vi "DAQ_TTC Meas Configure and Measure.vi"(0 "DAQmx Task In":refnum<k21>, 2 "Execution Option":T7, 5 "Range and Terminal Settings":T1={"Global Settings"={"Min Temp (deg C)"=0.0, "Max Temp (deg C)"=100.0, "Thermocouple Type"=10072, "CJC Temp (deg C)"=25.0, "Enable Autozero"=FALSE, "Auto Zero Mode"=10230}, "Specific Channel Settings"=[]} {"Specific Channel Settings"."Thermocouple Type" items=["J"=10072, "K"=10073, "N"=10077, "R"=10082, "S"=10085, "T"=10086, "B"=10047, "E"=10055]; "Global Settings"."Auto Zero Mode" items=["None"=10230, "Once"=10244, "Every Sample"=10164]; "Global Settings"."Thermocouple Type" items=["J"=10072, "K"=10073, "N"=10077, "R"=10082, "S"=10085, "T"=10086, "B"=10047, "E"=10055]; "Global Settings"."CJC Temp (deg C)" format="%.2f"; "Global Settings"."Min Temp (deg C)" format="%.2f"; "Global Settings"."Max Temp (deg C)" format="%.2f"}, 7 "Timing and Trigger Settings":T3={"Timing Settings"={"Sample Clock Source"="OnboardClock", "Sample Rate(Hz)"=100.0, "Number of Samples"=10, "Sample Timing Engine"=enum."Auto"}, "Trigger Settings"={"Trigger Type"=enum."No Trigger", "Digital Start Trigger Source"="", "Digital Start Trigger Edge"=10280}} {"Trigger Settings"."Digital Start Trigger Edge" items=["Rising"=10280, "Falling"=10171]; "Timing Settings"."Sample Rate(Hz)" format="%.2p"}, 11 "error in":errorcluster) -> (4 "DAQmx Task Out":refnum<k21>, 6 "Temperature Waveforms":waveform(dbl)[](graph), 8 "Temperature Measurements":T6 {"Average Temperature(K)" format="%.2p"; "Average Temperature(deg C)" format="%.2p"}, 10 "Acquisition Time (s)":dbl=0.1 format="%.2p", 15 "error out":errorcluster)   [LabVIEW 2021, in "DAQ_Temperature Thermocouple Measurement.lvlib"]
doc: "Configure, initiate and fetch temperature thermocouple measurements from the channels configured."
uses:
  DAQ_Temperature Thermocouple Measurement.lvlib
  Common/Typedefs/Execution Options - Measure.ctl
  Typedefs/Temperature Thermocouple Measurements.ctl
  Typedefs/Timing & Trigger Settings.ctl
  Typedefs/Timing Settings.ctl
  Typedefs/Trigger Settings.ctl
  Typedefs/Range and Terminal Settings.ctl
  Typedefs/Specific Channel Settings.ctl
  <vilib>/DAQmx/read.llb/DAQmx Read (Analog 1D Wfm NChan NSamp).vi
  <vilib>/DAQmx/configure/timing.llb/DAQmx Timing (Sample Clock).vi
  <vilib>/DAQmx/configure/trigger.llb/DAQmx Start Trigger (Digital Edge).vi
  <vilib>/DAQmx/miscellaneous.llb/DAQmx Fill In Error Info.vi
  <resource>/objmgr/daqmx.rc
panel:
  # "Outputs"
  # "Inputs"
  # "Physical Channel Name"
  # "Thermocouple Type"
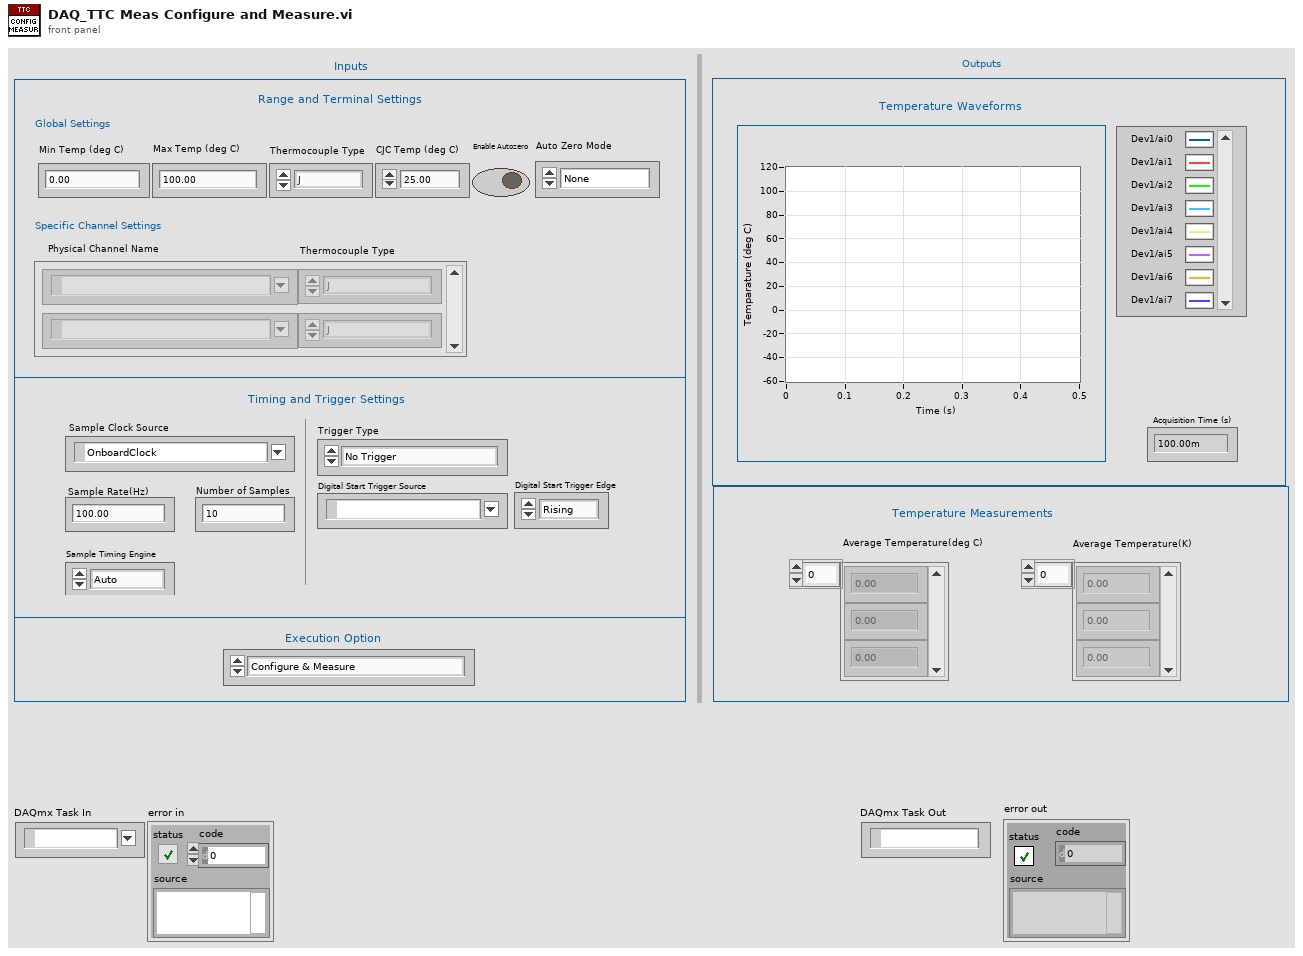
[diagram p1: front panel]
types:
  T1 = typedef "DAQ_Temperature Thermocouple Measurement.lvlib/Range and Terminal Settings.ctl" = cluster{"Global Settings":cluster{"Min Temp (deg C)":dbl, "Max Temp (deg C)":dbl, "Thermocouple Type":i32, "CJC Temp (deg C)":dbl, "Enable Autozero":bool, "Auto Zero Mode":i32}, "Specific Channel Settings":T2[]}
  T2 = typedef "DAQ_Temperature Thermocouple Measurement.lvlib/Specific Channel Settings.ctl" = cluster{"Physical Channel Name":tag, "Thermocouple Type":i32}
  T3 = typedef "DAQ_Temperature Thermocouple Measurement.lvlib/Timing & Trigger Settings.ctl" = cluster{"Timing Settings":T4, "Trigger Settings":T5}
  T4 = typedef "DAQ_Temperature Thermocouple Measurement.lvlib/Timing Settings.ctl" = cluster{"Sample Clock Source":tag, "Sample Rate(Hz)":dbl, "Number of Samples":i32, "Sample Timing Engine":enum16{"te0", "te1", "ai", "Auto"}}
  T5 = typedef "DAQ_Temperature Thermocouple Measurement.lvlib/Trigger Settings.ctl" = cluster{"Trigger Type":enum16{"No Trigger", "Digital Start"}, "Digital Start Trigger Source":tag, "Digital Start Trigger Edge":i32}
  T6 = typedef "DAQ_Temperature Thermocouple Measurement.lvlib/Temperature Thermocouple Measurements.ctl" = cluster{"Average Temperature(deg C)":dbl[], "Average Temperature(K)":dbl[]}
  T7 = typedef "Execution Options - Measure.ctl" = enum16{"Configure & Measure", "Configure only", "Measure only"}
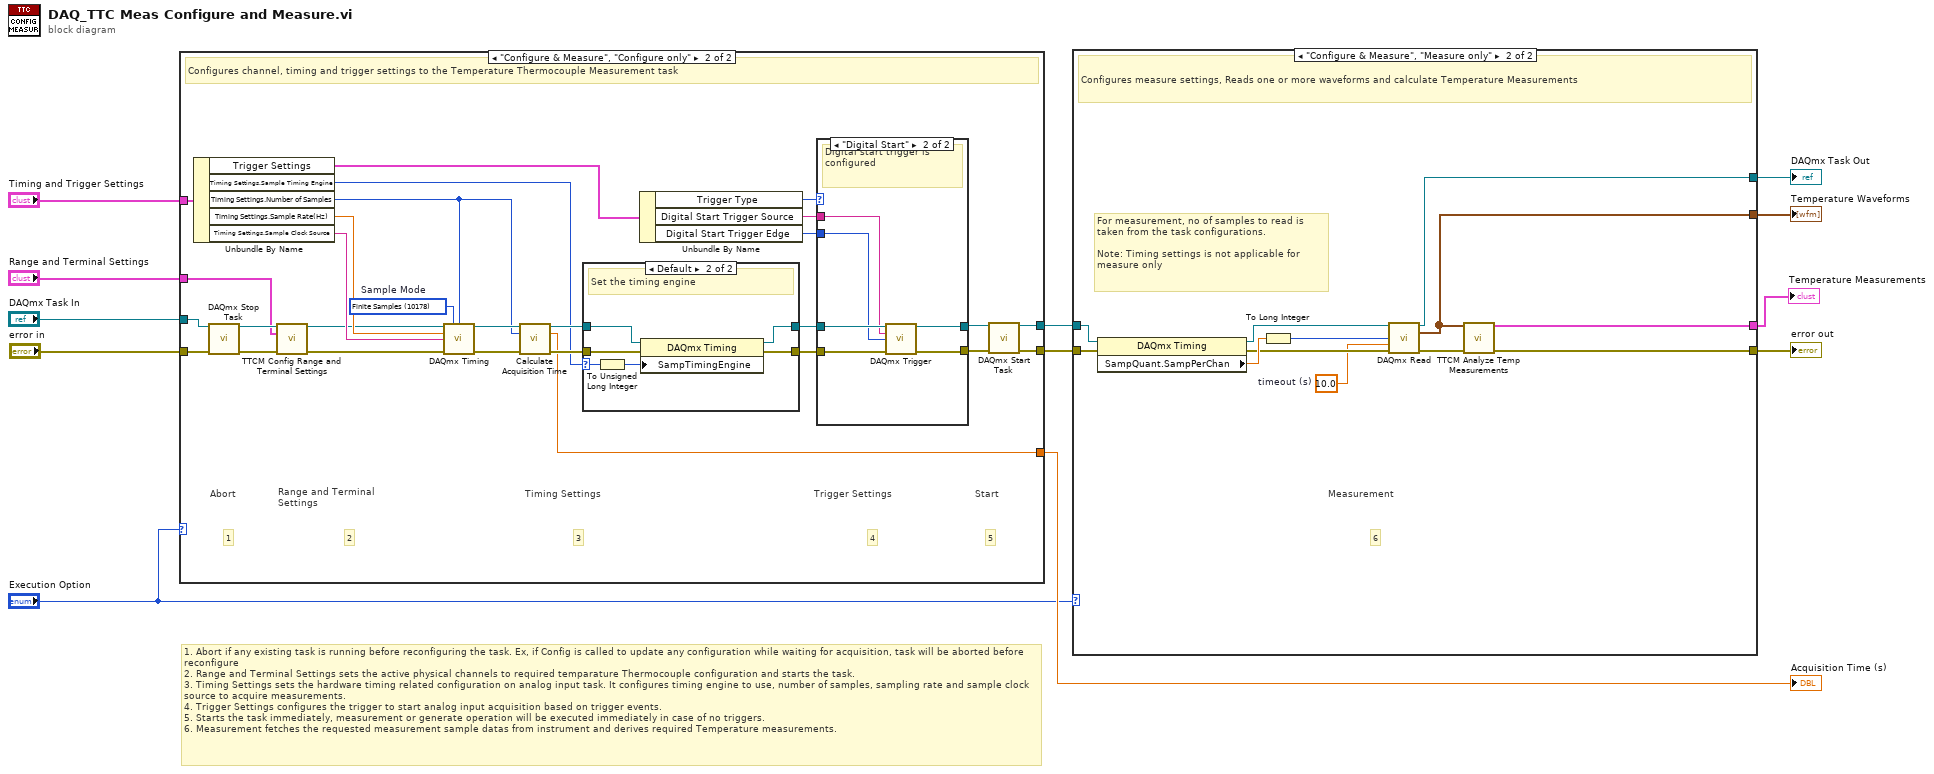
[diagram p0: block diagram]
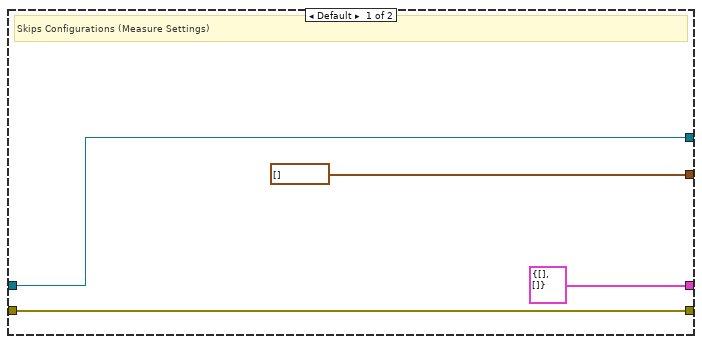
[diagram p5: hidden frame]
diagram:
  # "1. Abort if any existing task is running before reconfiguring the task. Ex, if Config is called to update any configuration while waiting for acquisition, task will be aborted before reconfigure\n2. Range and Terminal Settings sets the active physical channels to required temparature Thermocouple configuration and starts the task.\n3. Timing Settings sets the hardware timing related configuration on analog input task. It configures timing engine to use, number of samples, sampling rate and sample clock source to acquire measurements.\n4. Trigger Settings configures the trigger to start analog input acquisition based on trigger events.\n5. Starts the task immediately, measurement or generate operation will be executed immediately in case of no triggers.\n6. Measurement fetches the requested measurement sample datas from instrument and derives required Temperature measurements."
  n1 = case shown="\"Configure & Measure\", \"Configure only\"" "Execution Option" {
    tunnel: "error in" -> [w14 w19]
    tunnel: "DAQmx Task In" -> [w13 w21]
    tunnel: "Timing and Trigger Settings" -> [_ w36]
    tunnel: [w13 w17] -> w11
    tunnel: [w14 w30] -> w12
    tunnel: "Range and Terminal Settings" -> [_ w15]
    tunnel: [_ w16] -> w5
    frame Default {
      # "Skips Configurations (Channel, Timing and Trigger Settings)"
    }
    frame "Configure & Measure", "Configure only" {
      w40 = 10178 items=["Finite Samples"=10178, "Continuous Samples"=10123, "Hardware Timed Single Point"=12522]  # Sample Mode
      # "1"
      # "Abort"
      # "5"
      # "Start"
      # "4"
      # "3"
      # "2"
      # "Range and Terminal \nSettings"
      # "Trigger Settings"
      # "Timing Settings"
      # "Configures channel, timing and trigger settings to the Temperature Thermocouple Measurement task"
      n2 = Unbundle By Name(w36) -> ("Trigger Settings"=w23:T5, "Timing Settings.Sample Timing Engine"=w31:enum16{"te0", "te1", "ai", "Auto"}, "Timing Settings.Number of Samples"=w29:i32, "Timing Settings.Sample Rate(Hz)"=w37:dbl, "Timing Settings.Sample Clock Source"=w38:tag)
      n3 = call <vilib>:"DAQmx Stop Task.vi"("task/channels in"=w21, "error in"=w19) -> ("task out"=w22:refnum<k21>, "error out"=w20:errorcluster)  [unwired: 12 in]
      n4 = call "TTCM Config Range and Terminal Settings.vi"("DAQmx Task In"=w22, "Range and Terminal Settings"=w15, "error in (no error)"=w20) -> ("DAQmx Task Out"=w24:refnum<k21>, "error out"=w25:errorcluster)  [unwired: 11 in]
      n5 = call-poly <vilib>:"DAQmx Timing.vi"("task/channels in"=w24, "sample mode"=w40, "samples per channel"=w29, "rate"=w37, "source"=w38, "error in"=w25) -> ("task out"=w42:refnum<k21>, "error out"=w41:errorcluster)  [unwired: 8 in]
      n6 = call "Calculate Acquisition Time.vi"("Refnum in"=w42, "Number of Samples"=w29, "error in (no error)"=w41) -> ("Refnum out"=w33:refnum<k21>, "Acquisition Time Period (s)"=w16:dbl, "error out"=w39:errorcluster)  [unwired: 10 in]
      n7 = case shown="Default" w31 {
        selector: w31 -> [_ w46]
        tunnel: w39 -> [w44 w50]
        tunnel: [w44 w49] -> w34
        tunnel: w33 -> [w43 w48]
        tunnel: [w43 w47] -> w32
        frame "Auto" {
          # "Timing engine is auto-selected"
        }
        frame Default {
          # "Set the timing engine"
          n8 = To Unsigned Long Integer(number=w46) -> (unsigned 32bit integer=w45:u32)
          n9 = property class="DAQmx Timing"(reference=w48, error in=w50, "SampTimingEngine"=w45) -> (reference out=w47:refnum<k21>, error out=w49:errorcluster)
        }
      }
      n10 = Unbundle By Name(w23) -> ("Trigger Type"=w26:enum16{"No Trigger", "Digital Start"}, "Digital Start Trigger Source"=w28:tag, "Digital Start Trigger Edge"=w27:i32)
      n11 = case shown="\"Digital Start\"" w26 {
        tunnel: w32 -> [w52 w58]
        tunnel: w34 -> [w51 w57]
        tunnel: [w52 w56] -> w18
        tunnel: [w51 w55] -> w35
        tunnel: w28 -> [_ w54]
        tunnel: w27 -> [_ w53]
        frame Default {
          # "No Trigger settings has been configured"
        }
        frame "Digital Start" {
          # "Digital start trigger is configured"
          n12 = call-poly <vilib>:"DAQmx Trigger.vi"("task/channels in"=w58, "source"=w54, "edge"=w53, "error in"=w57) -> ("task out"=w56:refnum<k21>, "error out"=w55:errorcluster)  [unwired: 10 in]
        }
      }
      n13 = call <vilib>:"DAQmx Start Task.vi"("task/channels in"=w18, "error in"=w35) -> ("task out"=w17:refnum<k21>, "error out"=w30:errorcluster)  [unwired: 12 in]
    }
  }
  "Acquisition Time (s)" <- w5
  n14 = case shown="\"Configure & Measure\", \"Measure only\"" "Execution Option" {
    tunnel: w11 -> [w62 w71]
    tunnel: w12 -> [w61 w68]
    tunnel: [w62 w73] -> w10
    tunnel: [w61 w65] -> w8
    tunnel: [waveform(dbl)[] [] ("data") w64] -> w6
    tunnel: [T6 {"Average Temperature(deg C)"=[], "Average Temperature(K)"=[]} ("Measure Settings") w63] -> w3
    frame Default {
      # "Skips Configurations (Measure Settings)"
    }
    frame "Configure & Measure", "Measure only" {
      w66 = 10.0  # timeout (s)
      # "For measurement, no of samples to read is taken from the task configurations.\n\nNote: Timing settings is not applicable for measure only"
      # "6"
      # "Measurement"
      # "Configures measure settings, Reads one or more waveforms and calculate Temperature Measurements"
      n15 = property class="DAQmx Timing"(reference=w71, error in=w68) -> (reference out=w72:refnum<k21>, error out=w69:errorcluster, "SampQuant.SampPerChan"=w70:dbl)
      n16 = To Long Integer(number=w70) -> (32bit integer=w67:i32)
      n17 = call-poly <vilib>:"DAQmx Read.vi"("task/channels in"=w72, "number of samples per channel"=w67, "timeout"=w66, "error in"=w69) -> ("task out"=w73:refnum<k21>, "data"=w64:waveform(dbl)[], "error out"=w74:errorcluster)  [unwired: 9 in]
      n18 = call "TTCM Analyze Temp Measurements.vi"("Temperature Waveforms In"=w64, "error in (no error)"=w74) -> ("Measure Settings"=w63:T6, "error out"=w65:errorcluster)  [unwired: 12 in]
    }
  }
  "error out" <- w8
  "DAQmx Task Out" <- w10
  "Temperature Waveforms" <- w6
  "Temperature Measurements" <- w3
